vi "Handle GU Arrange List DClick Event.vi"(8 "error in":errorcluster, 9 "Coords":T1, 11 "CtlRef":refnum<vi>) -> (0 "error out":errorcluster, 2 "Item Names":string[][](array[string]))   [LabVIEW 2020, in "GUCalibration2.lvlib"]
uses:
  GUCalibration2.lvlib
  <vilib>/Utility/miscctls.llb/LVPoint32TypeDef.ctl
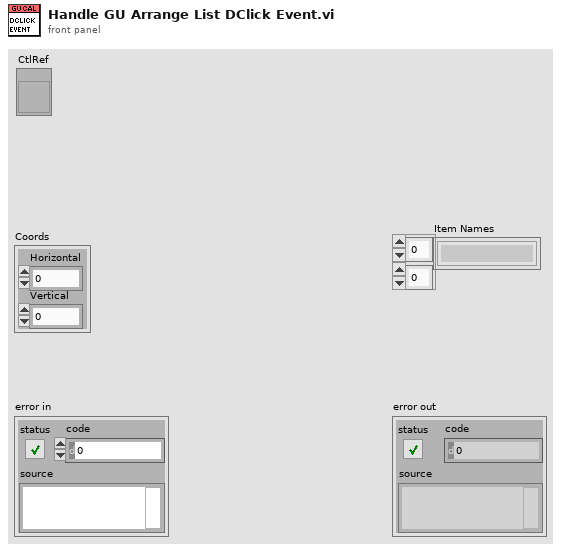
[diagram p1: front panel]
types:
  T1 = typedef "LVPoint32TypeDef.ctl" = cluster{"Horizontal":i32, "Vertical":i32}
  T2 = typedef "LVRowAndColumnTypeDef.ctl" = cluster{"Row":i32, "Column":i32}
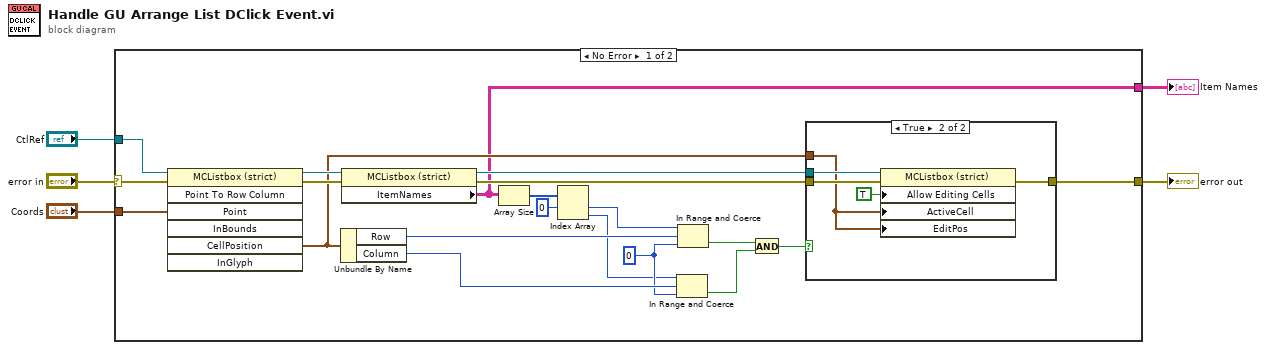
[diagram p0: block diagram]
diagram:
  n1 = case shown="No Error" "error in" {
    selector: "error in" -> [w7 w32]
    tunnel: "CtlRef" -> [w23 _]
    tunnel: "Coords" -> [w22 _]
    tunnel: [w19 w32] -> w3
    tunnel: [w6 _] -> w1
    frame No Error {
      w13 = 0 ("lower limit")
      n2 = invoke class="MCListbox (strict)" method="Point To Row Column"(reference=w23, error in=w7, "Point"=w22) -> (reference out=w21:refnum<vi>, error out=w20:errorcluster, "CellPosition"=w8:T2)  [unwired: 4 in, 4 out]
      n3 = Unbundle By Name(w8) -> ("Row"=w16:i32, "Column"=w14:i32)
      n4 = property class="MCListbox (strict)"(reference=w21, error in=w20) -> (reference out=w24:refnum<vi>, error out=w25:errorcluster, "ItemNames"=w6:string[][])
      n5 = Array Size(array=w6) -> (size(s)=w18:i32[])
      n6 = Index Array(array=w18, index #1=0 ("index")) -> (element #1=w15:i32, element #2=w12:i32)  [unwired: 1 in]
      n7 = In Range and Coerce(upper limit=w12, x=w14, lower limit=w13) -> (In Range?=w10:bool)  [unwired: 1 out]
      n8 = In Range and Coerce(upper limit=w15, x=w16, lower limit=w13) -> (In Range?=w11:bool)  [unwired: 1 out]
      n9 = And(x=w11, y=w10) -> (x .and. y?=w9:bool)
      n10 = case shown="True" w9 {
        tunnel: w25 -> [w26 w31]
        tunnel: w24 -> [_ w30]
        tunnel: [w26 w29] -> w19
        tunnel: w8 -> [_ w27]
        frame False {
        }
        frame True {
          n11 = property class="MCListbox (strict)"(reference=w30, error in=w31, "Allow Editing Cells"=TRUE, "ActiveCell"=w27, "EditPos"=w27) -> (error out=w29:errorcluster)  [unwired: 1 out]
        }
      }
    }
    frame Error {
    }
  }
  "error out" <- w3
  "Item Names" <- w1
